vi "Configuration Tool Main.vi"() -> ()   [LabVIEW 2014, in "Advanced Configuration Tool.lvlib"]
doc: "This is the main VI for the configuration editor."
uses:
  Advanced Configuration Tool.lvlib
  Controls/StateCluster.ctl
  <vilib>/NI/Configuration Framework/Repository/NISE_CEF_Repository.lvclass
  <vilib>/NI/Configuration Framework/Node/NodeRef.ctl
  <vilib>/NI/Configuration Framework/Node/NISE_CEF_Node.lvclass
  <vilib>/NI/Configuration Framework/Node/UserEventRef.ctl
  <vilib>/NI/Configuration Framework/Controls/EventCluster.ctl
  Controls/AddMessage.ctl
  Controls/MoveMessage.ctl
  <vilib>/Utility/error.llb/DialogType.ctl
  <vilib>/NI/Configuration Framework/hierarchy repo/NISE_CEF_HierarchyRepo.lvclass
  Classes/My System/My System.lvclass
  <vilib>/NI/AMC/Read Termination Message.vi
  <vilib>/NI/AMC/Create Single Message.vi
  <vilib>/NI/AMC/Update Message Routing Info.vi
  <vilib>/NI/AMC/Globals.vi
  <vilib>/NI/AMC/Send Message.vi
  <vilib>/NI/AMC/AMC.lvlib
  <vilib>/NI/Configuration Framework/NISE_CEF_TreeControl.lvlib
  <vilib>/NI/Configuration Framework/serializable configuration/NISE_CEF_serializable configuration.lvclass
panel:
  in  "View":string(tree)
  in  "Exit":bool
  # "Configurator"
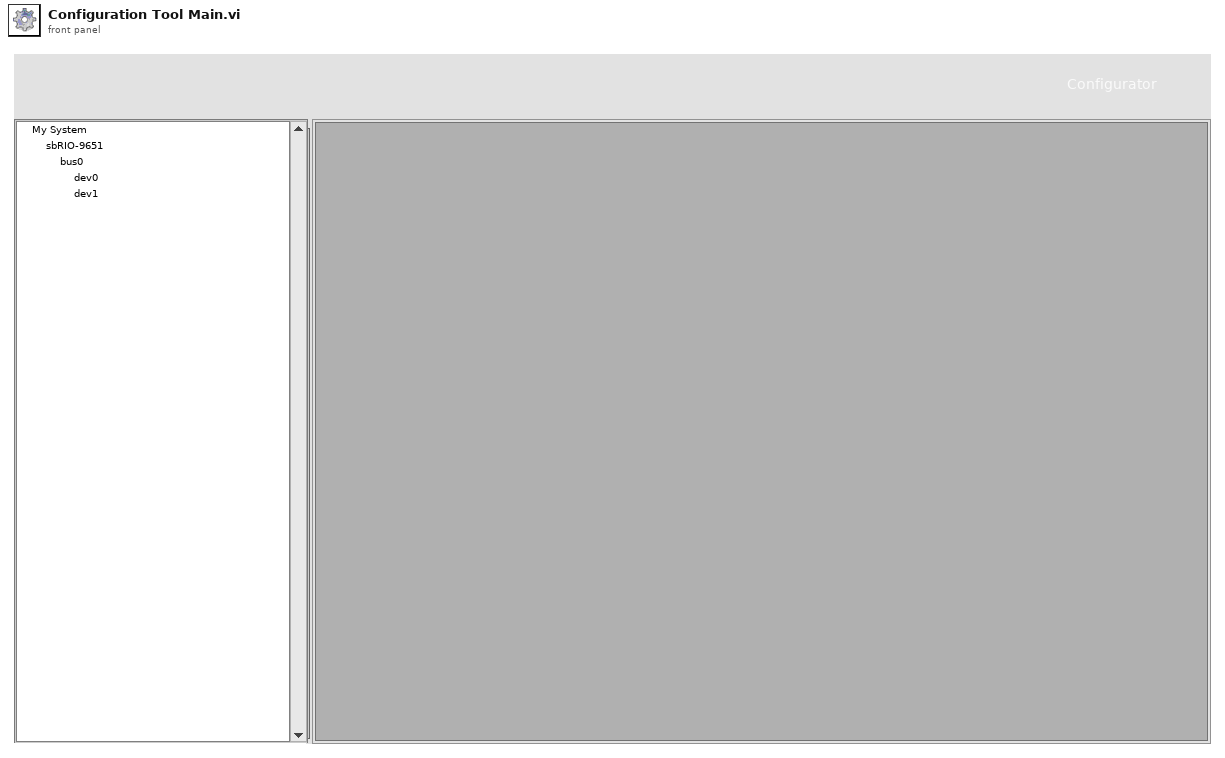
[diagram p1: front panel]
types:
  T1 = typedef "Advanced Configuration Tool.lvlib/StateCluster.ctl" = cluster{"repository":refnum<class "NISE_CEF_Repository.lvclass">, "root":T2, "unsaved changes":bool, "current path":path, "user event ref":T3, "glyph path":path, "classes path":path}
  T2 = typedef "NISE_CEF_Node.lvclass/NodeRef.ctl" = refnum<data-value>
  T3 = typedef "NISE_CEF_Node.lvclass/UserEventRef.ctl" = refnum<user-event>
  T4 = typedef "AMC.lvlib/Message Queue.ctl" = refnum<queue>
  T5 = typedef "Advanced Configuration Tool.lvlib/AddMessage.ctl" = cluster{"node type":string, "to add to":string}
  T6 = typedef "Advanced Configuration Tool.lvlib/MoveMessage.ctl" = cluster{"node ref":T2, "new parent":T2}
  T7 = typedef "NISE_CEF_TreeControl.lvlib/EventCluster.ctl" = cluster{"command":string, "data":string}
  T8 = typedef "Advanced Configuration Tool.lvlib/FilePaths.ctl" = cluster{"glyphs":path, "classes":path}
  T9 = typedef "DialogType.ctl" = u16
  T10 = typedef "NISE_CEF_Node.lvclass/Summary.ctl" = cluster{"ID":string, "parent ID":string, "node type":string, "text":string, "additional text":string, "glyph":string, "depth":i32}
  T11 = typedef "LVPoint32TypeDef.ctl" = cluster{"Horizontal":i32, "Vertical":i32}
  T12 = cluster{"data name":string, "drag data":variant}[]
  T13 = typedef "NISE_CEF_Node.lvclass/NodeMenuOptions.ctl" = cluster{"removable":bool, "movable":bool, "duplicate":bool}
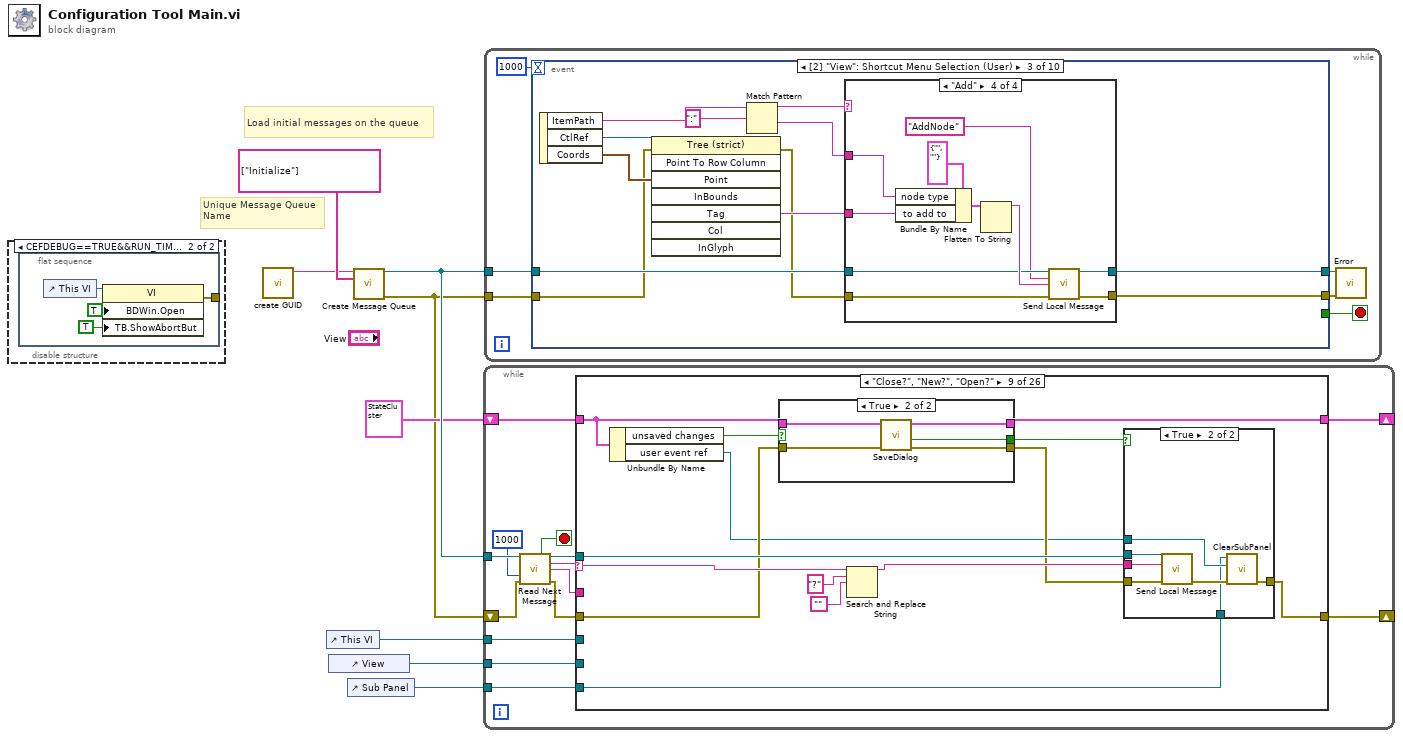
[diagram p0: block diagram]
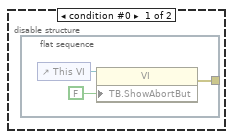
[diagram p2: hidden frame]
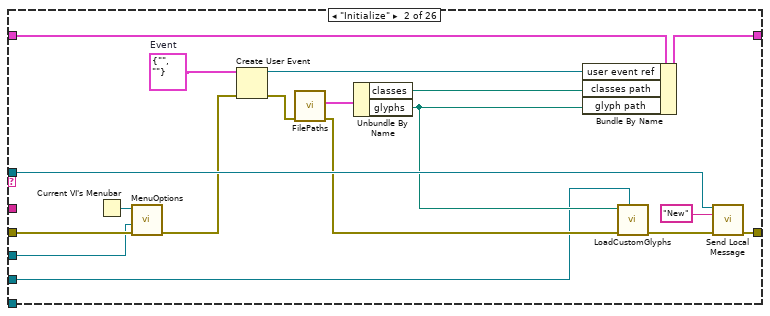
[diagram p4: hidden frame]
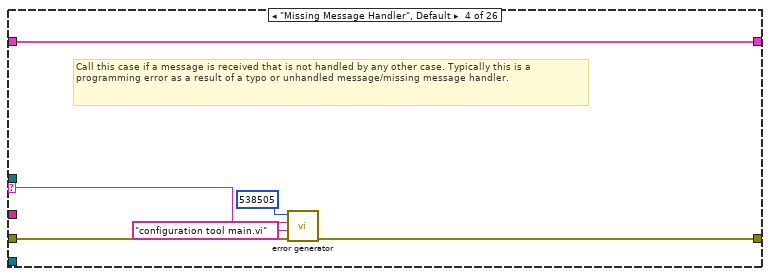
[diagram p6: hidden frame]
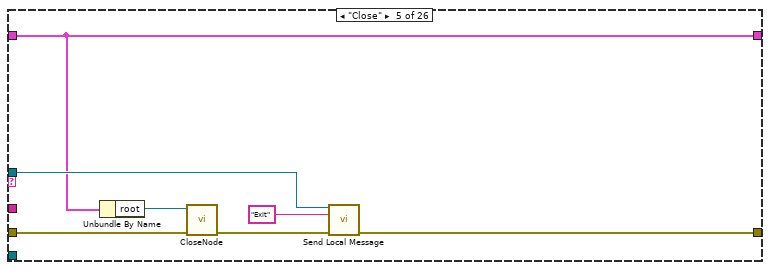
[diagram p7: hidden frame]
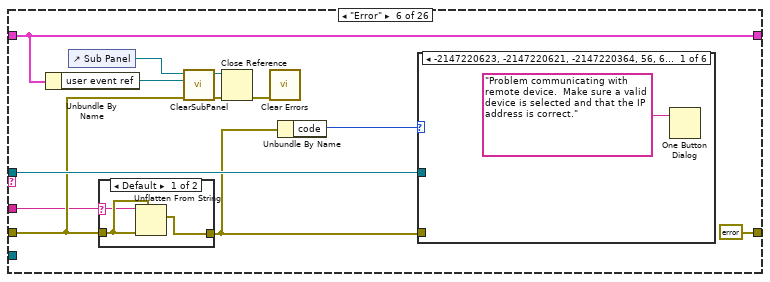
[diagram p8: hidden frame]
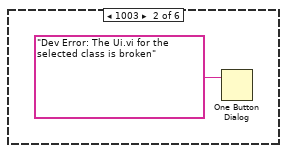
[diagram p10: hidden frame]
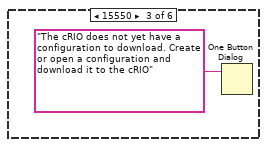
[diagram p11: hidden frame]
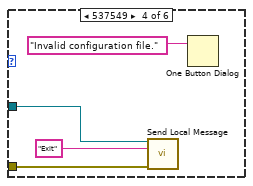
[diagram p12: hidden frame]
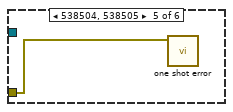
[diagram p13: hidden frame]
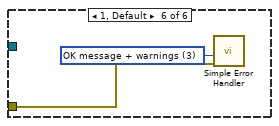
[diagram p14: hidden frame]
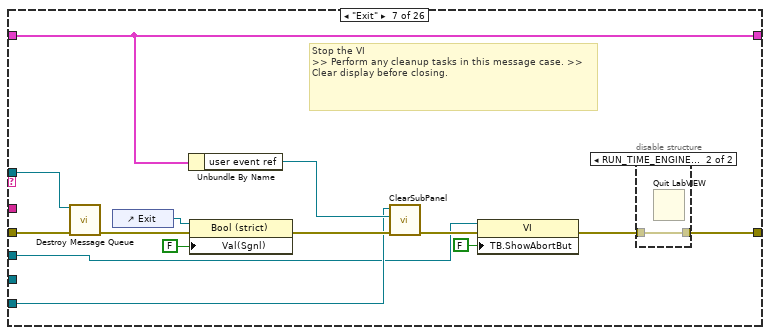
[diagram p15: hidden frame]
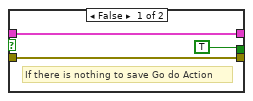
[diagram p18: hidden frame]
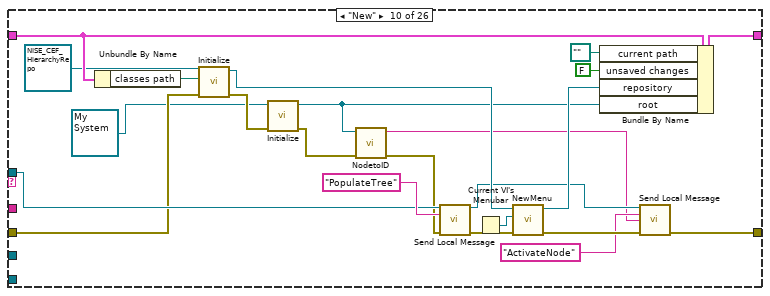
[diagram p20: hidden frame]
diagram:
  # "Unique Message Queue Name"
  # "Load initial messages on the queue"
  n1 = disable-structure shown="CEFDEBUG==TRUE&&RUN_TIME_ENGINE==False" {
    frame condition #0 {
      n2 = flat-sequence {
        tunnel: [w9] -> _
        frame #0 {
          n3 = control-ref of="This VI"() -> (w10:refnum<vi>)
          n4 = property class="VI"(reference=w10, "TB.ShowAbortBut"=FALSE ("Tool Bar:Show Abort Button")) -> (error out=w9:errorcluster)  [unwired: 1 in, 1 out]
        }
      }
    }
    frame condition #1 (active) {
      n5 = flat-sequence {
        tunnel: [w14] -> _
        frame #0 {
          n6 = control-ref of="This VI"() -> (w15:refnum<vi>)
          n7 = property class="VI"(reference=w15, "BDWin.Open"=TRUE ("Block Diagram Window:Open"), "TB.ShowAbortBut"=TRUE ("Tool Bar:Show Abort Button")) -> (error out=w14:errorcluster)  [unwired: 1 in, 1 out]
        }
      }
    }
  }
  n8 = call <vilib>:"create GUID.vi"() -> ("uuid"=w1:string)  [unwired: 11 in]
  n9 = control-ref of="This VI"() -> (w4:refnum<vi>)
  n10 = control-ref of="View"() -> (w3:refnum<vi>)
  n11 = control-ref of="Sub Panel"() -> (w2:refnum<vi>)
  n12 = call <vilib>:"Create Message Queue.vi"("message queue name"=w1, "initial message names"=string[] ["Initialize"]) -> ("message queue out"=w7:T4, "error out"=w5:errorcluster)  [unwired: 12 in]
  n13 = while "Message Processor" {
    shift-right: [w25] -> _
    shift-left: w5 -> [w24]
    tunnel: w7 -> [w23]
    shift-right: [w21] -> _
    shift-left: T1 {"repository"=refnum, "root"=refnum, "unsaved changes"=FALSE, "current path"=path "", "user event ref"=refnum, "glyph path"=path "", "classes path"=path ""} -> [w20]
    tunnel: w4 -> [w18]
    tunnel: w3 -> [w17]
    tunnel: w2 -> [w16]
    stop <- w29 stop-if-true
    n14 = call <vilib>:"Read Next Message.vi"("message queue in"=w23, "timeout (1 ms)"=1000, "error in"=w24) -> ("exit process?"=w29:bool, "message queue out"=w19:T4, "message name"=w28:string, "message value"=w27:string, "error out"=w26:errorcluster)  [unwired: 5 in, 3 out]
    n15 = case shown="\"Close?\", \"New?\", \"Open?\"" w28 {
      selector: w28 -> [_ _ _ w54 _ _ _ _ w118 _ _ _ _ _ _ _ _ _ _ w366 _ _ _ _ _ _]
      tunnel: w27 -> [_ _ _ _ _ w65 _ _ _ _ _ _ _ w240 w272 _ w300 w332 w346 w364 w404 w428 _ _ w471 w493]
      tunnel: w26 -> [w31 w49 w51 w56 w59 w68 w104 w108 w111 w155 w166 w206 w232 w247 w273 w290 w301 w322 w345 w369 w406 w427 w452 w461 w470 w491]
      tunnel: [w31 w45 w51 w55 w63 errorcluster {"status"=FALSE, "code"=0, "source"=""} ("error out") w97 w108 w122 w146 w162 w210 w234 w244 w260 w290 w304 w324 w349 w372 w410 w424 w447 w456 w467 w486] -> w25
      tunnel: [w30 w40 w50 w57 w61 w73 w96 w107 w113 w159 w167 w213 w233 w241 w269 w289 w307 w315 w342 w373 w408 w421 w454 w460 w465 w482] -> w21
      tunnel: w20 -> [w30 w41 w50 w57 w61 w73 w96 w107 w114 w158 w168 w208 w231 w242 w270 w289 w303 w320 w350 w373 w409 w429 w454 w460 w465 w494]
      tunnel: w19 -> [_ w44 _ _ w62 w76 w103 _ w121 w160 w164 w209 _ w243 w265 _ w291 _ _ w367 _ _ _ _ w466 w485]
      tunnel: w18 -> [_ w32 _ _ _ _ w92 _ _ _ _ _ _ _ _ _ _ _ _ _ _ _ w439 _ _ _]
      tunnel: w17 -> [_ w33 _ _ _ _ _ _ _ _ _ _ _ _ _ _ _ w316 w343 w361 w401 w422 w440 _ _ _]
      tunnel: w16 -> [_ _ _ _ _ _ w94 _ w109 _ _ _ _ _ _ _ _ _ _ _ _ _ w437 w455 w462 _]
      frame "------------Generic Operations------------" {
        # "Dummy case to add a seperation in the Case Structure menu"
      }
      frame "Initialize" {
        w35 = T7 {"command"="", "data"=""}  # Event
        n16 = Current VI's Menubar() -> (w48:refnum<k9>)
        n17 = call "MenuOptions.vi"("error in"=w49, "VI ref"=w32, "menu ref in"=w48) -> ("error out"=w39:errorcluster)  [unwired: 7 in, 1 out]
        n18 = Create User Event(user event datatype=w35, error in=w39) -> (user event=w34:refnum<user-event>, error out=w38:errorcluster)
        n19 = call "FilePaths.vi"("error in"=w38) -> ("error out"=w43:errorcluster, "paths"=w42:T8)  [unwired: 9 in]
        n20 = Unbundle By Name(w42) -> ("classes"=w37:path, "glyphs"=w36:path)
        n21 = Bundle By Name(cluster=w41, "user event ref"=w34, "classes path"=w37, "glyph path"=w36) -> (w40:T1)
        n22 = call <vilib>:"LoadCustomGlyphs.vi"("tree ref"=w33, "error in"=w43, "glyph directory"=w36) -> ("error out"=w46:errorcluster)  [unwired: 8 in]
        n23 = call <vilib>:"Send Local Message.vi"("message queue in"=w44, "message name"="New" ("Message Name"), "error in"=w46) -> ("error out"=w45:errorcluster)  [unwired: 10 in, 2 out]
      }
      frame "", "Idle" {
      }
      frame "Missing Message Handler", Default {
        # "Call this case if a message is received that is not handled by any other case. Typically this is a programming error as a result of a typo or unhandled message/missing message handler."
        n24 = call <vilib>:"error generator.vi"("error in"=w56, "source"="configuration tool main.vi", "append error message"=w54, "error code (0)"=538505) -> ("error out"=w55:errorcluster)  [unwired: 5 in]
      }
      frame "Close" {
        n25 = Unbundle By Name(w61) -> ("root"=w60:T2)
        n26 = call <vilib>:"CloseNode.vi"("error in"=w59, "node ref"=w60) -> ("error out"=w58:errorcluster)  [unwired: 9 in]
        n27 = call <vilib>:"Send Local Message.vi"("message queue in"=w62, "message name"="Exit", "error in"=w58) -> ("error out"=w63:errorcluster)  [unwired: 10 in, 2 out]
      }
      frame "Error" {
        n28 = Unbundle By Name(w73) -> ("user event ref"=w71:T3)
        n29 = control-ref of="Sub Panel"() -> (w72:refnum<vi>)
        n30 = case shown="Default" w65 {
          selector: w65 -> [w78 _]
          tunnel: w68 -> [w79 w80]
          tunnel: [w77 w80] -> w67
          frame Default {
            n31 = Unflatten From String(type=w79, binary string=w78, error in (no error)=w79) -> (value=w77:errorcluster)  [unwired: 2 in, 2 out]
          }
          frame "" {
          }
        }
        n32 = call <vilib>:"ClearSubPanel.vi"("error in"=w68, "user event ref"=w71, "sub panel ref in"=w72) -> ("error out"=w70:errorcluster, "sub panel ref out"=w69:refnum<vi>)  [unwired: 7 in]
        n33 = Close Reference(reference=w69, error in (no error)=w70) -> (error out=w66:errorcluster)
        n34 = call <vilib>:"Clear Errors.vi"("error in (no error)"=w66) -> ()  [unwired: 5 in, 2 out]
        n35 = Unbundle By Name(w67) -> ("code"=w74:i32)
        n36 = case shown="-2147220623, -2147220621, -2147220364, 56, 63" w74 {
          tunnel: w76 -> [_ _ _ w86 _ _]
          tunnel: w67 -> [_ _ _ w85 w88 w90]
          frame -2147220623, -2147220621, -2147220364, 56, 63 {
            n37 = One Button Dialog(message="Problem communicating with remote device.  Make sure a valid device is selected and that the IP address is correct.") -> ()  [unwired: 1 in, 1 out]
          }
          frame 1003 {
            n38 = One Button Dialog(message="Dev Error: The Ui.vi for the selected class is broken") -> ()  [unwired: 1 in, 1 out]
          }
          frame 15550 {
            n39 = One Button Dialog(message="The cRIO does not yet have a configuration to download. Create or open a configuration and download it to the cRIO") -> ()  [unwired: 1 in, 1 out]
          }
          frame 537549 {
            n40 = call <vilib>:"Send Local Message.vi"("message queue in"=w86, "message name"="Exit", "error in"=w85) -> ()  [unwired: 10 in, 3 out]
            n41 = One Button Dialog(message="Invalid configuration file.") -> ()  [unwired: 1 in, 1 out]
          }
          frame 538504, 538505 {
            n42 = call <vilib>:"one shot error.vi"("error in"=w88) -> ()  [unwired: 11 in]
          }
          frame 1, Default {
            w89 = T9 3 items=["no dialog", "OK message", "continue or stop message", "OK message + warnings", "continue/stop + warnings"] ("type of dialog (OK msg:1)")
            n43 = call <vilib>:"Simple Error Handler.vi"("type of dialog (OK msg:1)"=w89, "error in (no error)"=w90) -> ()  [unwired: 8 out]
          }
        }
      }
      frame "Exit" {
        # "Stop the VI                                                                             >> Perform any cleanup tasks in this message case. >> Clear display before closing."
        n44 = call <vilib>:"Destroy Message Queue.vi"("message queue in"=w103, "error in"=w104) -> ("error out"=w100:errorcluster)  [unwired: 11 in, 2 out]
        n45 = control-ref of="Exit"() -> (w102:refnum<vi>)
        n46 = Unbundle By Name(w96) -> ("user event ref"=w95:T3)
        n47 = property class="Bool (strict)"(reference=w102, error in=w100, "Val(Sgnl)"=FALSE ("Exit")) -> (error out=w99:errorcluster)  [unwired: 1 out]
        n48 = call <vilib>:"ClearSubPanel.vi"("error in"=w99, "user event ref"=w95, "sub panel ref in"=w94) -> ("error out"=w98:errorcluster)  [unwired: 7 in, 1 out]
        n49 = property class="VI"(reference=w92, error in=w98, "TB.ShowAbortBut"=FALSE ("Tool Bar:Show Abort Button")) -> (error out=w93:errorcluster)  [unwired: 1 out]
        n50 = disable-structure shown="RUN_TIME_ENGINE==True" {
          disable-tunnel: [w105 w106] -> w97
          disable-tunnel: w93 -> [w105 w106]
          frame condition #0 (active) {
          }
          frame condition #1 {
            n51 = Quit LabVIEW() -> ()  [unwired: 1 in]
          }
        }
      }
      frame "------------Menu Operations--------------" {
        # "Dummy case to add a seperation in the Case Structure menu"
      }
      frame "Close?", "New?", "Open?" {
        n52 = Unbundle By Name(w114) -> ("unsaved changes"=w116:bool, "user event ref"=w110:T3)
        n53 = case shown="True" w116 {
          tunnel: [TRUE ("SaveFlag") w130] -> w115
          tunnel: w114 -> [w124 w129]
          tunnel: [w124 w128] -> w113
          tunnel: w111 -> [w123 w127]
          tunnel: [w123 w126] -> w112
          frame False {
            # "If there is nothing to save Go do Action"
          }
          frame True {
            n54 = call "SaveDialog.vi"("error in"=w127, "state in"=w129) -> ("error out"=w126:errorcluster, "new"=w130:bool, "state out"=w128:T1)  [unwired: 7 in]
          }
        }
        n55 = Search and Replace String(input string=w118, search string="?", replace string="") -> (result string=w117:string)  [unwired: 5 in, 3 out]
        n56 = case shown="True" w115 {
          tunnel: w112 -> [w131 w138]
          tunnel: [w131 w134] -> w122
          tunnel: w121 -> [_ w137]
          tunnel: w117 -> [_ w136]
          tunnel: w110 -> [_ w133]
          tunnel: w109 -> [_ w132]
          frame False {
          }
          frame True {
            n57 = call <vilib>:"Send Local Message.vi"("message queue in"=w137, "message name"=w136, "error in"=w138) -> ("error out"=w135:errorcluster)  [unwired: 10 in, 2 out]
            n58 = call <vilib>:"ClearSubPanel.vi"("error in"=w135, "user event ref"=w133, "sub panel ref in"=w132) -> ("error out"=w134:errorcluster)  [unwired: 7 in, 1 out]
          }
        }
      }
      frame "New" {
        n59 = Unbundle By Name(w158) -> ("classes path"=w157:path)
        n60 = call-dynamic "Initialize.vi"("error in"=w155, "path"=w157, "repository in"=refnum<class "NISE_CEF_HierarchyRepo.lvclass"> refnum ("NISE_CEF_HierarchyRepo.lvclass")) -> ("error out"=w156:errorcluster, "repository out"=w149:refnum<class "NISE_CEF_HierarchyRepo.lvclass">)  [unwired: 7 in]
        n61 = call-dynamic "Initialize.vi"("error in"=w156, "node in"=refnum<class "My System.lvclass"> refnum ("My System.lvclass")) -> ("error out"=w143:errorcluster, "data value reference"=w144:T2)  [unwired: 7 in, 1 out]
        n62 = call <vilib>:"NodetoID.vi"("error in"=w143, "node ref"=w144) -> ("error out"=w142:errorcluster, "ID"=w140:string)  [unwired: 8 in]
        n63 = call <vilib>:"Send Local Message.vi"("message queue in"=w160, "message name"="PopulateTree", "error in"=w142) -> ("message queue out"=w145:T4, "error out"=w151:errorcluster)  [unwired: 10 in, 1 out]
        n64 = Current VI's Menubar() -> (w150:refnum<k9>)
        n65 = call <vilib>:"NewMenu.vi"("error in"=w151, "menu ref in"=w150, "NISE_CEF_Repository in"=w149) -> ("error out"=w147:errorcluster, "NISE_CEF_Repository out"=w148:refnum<class "NISE_CEF_HierarchyRepo.lvclass">)  [unwired: 6 in, 1 out]
        n66 = Bundle By Name(cluster=w158, "current path"=path "", "unsaved changes"=FALSE, "repository"=w148, "root"=w144) -> (w159:T1)
        n67 = call <vilib>:"Send Local Message.vi"("message queue in"=w145, "message name"="ActivateNode", "message value"=w140, "error in"=w147) -> ("error out"=w146:errorcluster)  [unwired: 9 in, 2 out]
      }
      frame "Open" {
        n68 = in-place {
          in-place-border: w166 -> [w174]
          in-place-border: [w173] -> w163
          n69 = in-place-cluster #1(w168) -> ("current path"=w170:path, "repository"=w182:refnum<class "NISE_CEF_Repository.lvclass">, "root"=w178:T2)  [unwired: 1 out]
          n70 = call "generate default path.vi"("current file path"=w170) -> ("browse path"=w169:path)  [unwired: 10 in]
          n71 = call "FileDialog.vi"("error in"=w174, "start path"=w169) -> ("error out"=w175:errorcluster, "cancelled"=w176:bool, "selected path"=w172:path)  [unwired: 7 in]
          n72 = Compound Arithmetic op=OR(invert w176) -> (w177:bool)
          n73 = case shown="True" w177 {
            tunnel: w182 -> [w183 w195]
            tunnel: [w183 w193] -> w180
            tunnel: [w184 w191] -> w173
            tunnel: [w185 w190] -> w179
            tunnel: w172 -> [_ w188]
            tunnel: w175 -> [w184 w187]
            tunnel: w178 -> [w185 w186]
            frame False {
            }
            frame True {
              n74 = call-dynamic "Open.vi"("error in"=w187, "file path"=w188, "repository in"=w195) -> ("error out"=w192:errorcluster, "invalid?"=w189:bool, "repository out"=w194:refnum<class "NISE_CEF_Repository.lvclass">)  [unwired: 6 in]
              n75 = case shown="False" w189 {
                tunnel: w194 -> [w200 w203]
                tunnel: [w199 w203] -> w193
                tunnel: w192 -> [w198 w202]
                tunnel: [w197 w202] -> w191
                tunnel: [w196 w201] -> w190
                tunnel: w186 -> [_ w201]
                frame False {
                  n76 = call-dynamic "WriteTree.vi"("error in"=w198, "repository in"=w200) -> ("error out"=w197:errorcluster, "root"=w196:T2, "repository out"=w199:refnum<class "NISE_CEF_Repository.lvclass">)  [unwired: 7 in]
                }
                frame True {
                }
              }
            }
          }
          n77 = Select(t=w170, s=w173, f=w172) -> (s? t:f=w171:path)
          n78 = in-place-cluster #1("current path"=w171, "unsaved changes"=FALSE ("SaveFlag"), "repository"=w180, "root"=w179) -> (w167:T1)
        }
        n79 = call <vilib>:"Send Local Message.vi"("message queue in"=w164, "message name"="PopulateTree", "error in"=w163) -> ("error out"=w162:errorcluster)  [unwired: 10 in, 2 out]
      }
      frame "Save" {
        n80 = in-place {
          in-place-border: w206 -> [w218]
          in-place-border: [w217] -> w205
          in-place-border: [w215] -> w204
          n81 = in-place-cluster #2(w208) -> ("current path"=w216:path, "root"=w219:T2, "repository"=w220:refnum<class "NISE_CEF_Repository.lvclass">)
          n82 = Empty String/Path?(string/path=w216) -> (empty?=w215:bool)
          n83 = call-dynamic "ReadTree.vi"("error in"=w218, "root"=w219, "repository in"=w220) -> ("error out"=w217:errorcluster, "repository out"=w214:refnum<class "NISE_CEF_Repository.lvclass">)  [unwired: 7 in]
          n84 = in-place-cluster #2("current path"=w216, "root"=w219, "repository"=w214) -> (w207:T1)
        }
        n85 = case shown="True" w204 {
          tunnel: w207 -> [w224 w226]
          tunnel: [w223 w225] -> w213
          tunnel: [w222 w227] -> w211
          tunnel: w205 -> [w221 w228]
          frame False {
            n86 = call "Save.vi"("error in"=w221, "state in"=w224) -> ("error out"=w222:errorcluster, "state out"=w223:T1)  [unwired: 8 in]
          }
          frame True {
            # "Empty path use Dialog"
            n87 = call "SaveAs.vi"("error in"=w228, "state in"=w226) -> ("error out"=w227:errorcluster, "state out"=w225:T1)  [unwired: 7 in, 1 out]
          }
        }
        n88 = call <vilib>:"Send Local Message.vi"("message queue in"=w209, "message name"="PopulateTree", "error in"=w211) -> ("error out"=w210:errorcluster)  [unwired: 10 in, 2 out]
      }
      frame "SaveAs" {
        n89 = in-place {
          in-place-border: w232 -> [w236]
          in-place-border: [w235] -> w230
          n90 = in-place-cluster #3(w231) -> ("root"=w237:T2, "repository"=w239:refnum<class "NISE_CEF_Repository.lvclass">)
          n91 = call-dynamic "ReadTree.vi"("error in"=w236, "root"=w237, "repository in"=w239) -> ("error out"=w235:errorcluster, "repository out"=w238:refnum<class "NISE_CEF_Repository.lvclass">)  [unwired: 7 in]
          n92 = in-place-cluster #3("root"=w237, "repository"=w238) -> (w229:T1)
        }
        n93 = call "SaveAs.vi"("error in"=w230, "state in"=w229) -> ("error out"=w234:errorcluster, "state out"=w233:T1)  [unwired: 7 in, 1 out]
      }
      frame "Custom View" {
        n94 = in-place {
          in-place-border: w247 -> [w258]
          in-place-border: [w257] -> w245
          in-place-border: w240 -> [w248]
          n95 = in-place-cluster #4(w242) -> ("repository"=w252:refnum<class "NISE_CEF_Repository.lvclass">, "root"=w251:T2)
          n96 = call-dynamic "ReadTree.vi"("error in"=w258, "root"=w251, "repository in"=w252) -> ("error out"=w255:errorcluster, "repository out"=w254:refnum<class "NISE_CEF_Repository.lvclass">)  [unwired: 7 in]
          n97 = call-dynamic "CustomView.vi"("error in"=w255, "view name"=w248, "repository in"=w254) -> ("error out"=w256:errorcluster, "repository out"=w253:refnum<class "NISE_CEF_Repository.lvclass">)  [unwired: 7 in]
          n98 = call-dynamic "WriteTree.vi"("error in"=w256, "repository in"=w253) -> ("error out"=w257:errorcluster, "root"=w249:T2, "repository out"=w250:refnum<class "NISE_CEF_Repository.lvclass">)  [unwired: 7 in]
          n99 = in-place-cluster #4("repository"=w250, "root"=w249) -> (w241:T1)
        }
        n100 = call <vilib>:"Send Local Message.vi"("message queue in"=w243, "message name"="PopulateTree", "error in"=w245) -> ("error out"=w244:errorcluster)  [unwired: 10 in, 2 out]
      }
      frame "CustomFileMenu" {
        n101 = Unflatten From String(type=cluster{"ItemTag":string, string} {"ItemTag"="", ""} ("output cluster"), binary string=w272, error in (no error)=w273) -> (value=w259:cluster{"ItemTag":string, string}, error out=w268:errorcluster)  [unwired: 2 in, 1 out]
        n102 = Unbundle By Name(w270) -> ("repository"=w267:refnum<class "NISE_CEF_Repository.lvclass">)
        n103 = Unbundle(w259) -> ("ItemTag"=w264:string, w263:string)
        n104 = call-dynamic "HandleMenu.vi"("message queue"=w265, "error in"=w268, "Item Path"=w263, "ItemTag"=w264, "NISE_CEF_Repository in"=w267) -> ("error out"=w262:errorcluster, "handled?"=w261:bool, "NISE_CEF_Repository out"=w266:refnum<class "NISE_CEF_Repository.lvclass">)  [unwired: 4 in]
        n105 = case shown="False" w261 {
          tunnel: w262 -> [w277 w288]
          tunnel: [w278 w288] -> w260
          tunnel: w259 -> [w276 _]
          frame False {
            n106 = Unbundle(w276) -> ("ItemTag"=w275:string, w274:string)
            n107 = disable-structure shown="Default" {
              disable-tunnel: w277 -> [w284 w287]
              disable-tunnel: [w283 w287] -> w278
              disable-tunnel: w274 -> [w282 _]
              disable-tunnel: w275 -> [w281 _]
              frame condition #0 (active) {
                n108 = Concatenate Strings(w281, "::" ("string"), w282) -> (w280:string)
                n109 = call <vilib>:"error generator.vi"("error in"=w284, "source"="configuration tool main.vi", "append error message"=w280, "error code (0)"=538506) -> ("error out"=w283:errorcluster)  [unwired: 5 in]
              }
              frame condition #1 {
              }
            }
          }
          frame True {
          }
        }
        n110 = Bundle By Name(cluster=w270, "repository"=w266) -> (w269:T1)
      }
      frame "-------TreeControl Operations-----------" {
        # "Dummy case to add a seperation in the Case Structure menu"
      }
      frame "Select Target" {
        n111 = in-place {
          in-place-border: w301 -> [w311]
          in-place-border: w300 -> [w310]
          in-place-border: [w309] -> w297
          in-place-border: [w308] -> w298
          n112 = in-place-cluster #5(w303) -> ("repository"=w313:refnum<class "NISE_CEF_Repository.lvclass">)
          n113 = call-dynamic "GetClassPath.vi"("error in"=w311, "class name"=w310, "Repository in"=w313) -> ("error out"=w309:errorcluster, "class path"=w308:path, "Repository out"=w312:refnum<class "NISE_CEF_Repository.lvclass">)  [unwired: 6 in]
          n114 = in-place-cluster #5("repository"=w312) -> (w302:T1)
        }
        n115 = call <vilib>:"Get LV Class Default Value.vi"("error in (no error)"=w297, "class path"=w298) -> ("error out"=w296:errorcluster, "object"=w299:refnum<class>)  [unwired: 8 in]
        n116 = To More Specific Class(target class=refnum<class "NISE_CEF_Node.lvclass"> refnum ("Node.lvclass"), reference=w299, error in=w296) -> (specific class reference=w294:refnum<class "NISE_CEF_Node.lvclass">, error out=w293:errorcluster)
        n117 = call-dynamic "Initialize.vi"("error in"=w293, "node in"=w294) -> ("error out"=w292:errorcluster, "data value reference"=w306:T2)  [unwired: 7 in, 1 out]
        n118 = Bundle By Name(cluster=w302, "root"=w306) -> (w307:T1)
        n119 = call <vilib>:"Send Local Message.vi"("message queue in"=w291, "message name"="PopulateTree", "error in"=w292) -> ("error out"=w304:errorcluster)  [unwired: 10 in, 2 out]
      }
      frame "AddNode" {
        n120 = Unflatten From String(type=T5 {"node type"="", "to add to"=""} ("input cluster"), binary string=w332) -> (value=w330:T5)  [unwired: 3 in, 2 out]
        n121 = Unbundle By Name(w330) -> ("to add to"=w327:string, "node type"=w318:string)
        n122 = in-place {
          in-place-border: w322 -> [w338]
          in-place-border: [w337] -> w321
          in-place-border: w318 -> [w336]
          in-place-border: [w335] -> w317
          n123 = in-place-cluster #6(w320) -> ("repository"=w340:refnum<class "NISE_CEF_Repository.lvclass">)
          n124 = call-dynamic "GetClassPath.vi"("error in"=w338, "class name"=w336, "Repository in"=w340) -> ("error out"=w337:errorcluster, "class path"=w335:path, "Repository out"=w339:refnum<class "NISE_CEF_Repository.lvclass">)  [unwired: 6 in]
          n125 = in-place-cluster #6("repository"=w339) -> (w319:T1)
        }
        n126 = call <vilib>:"Get LV Class Default Value.vi"("error in (no error)"=w321, "class path"=w317) -> ("error out"=w333:errorcluster, "object"=w334:refnum<class>)  [unwired: 8 in]
        n127 = To More Specific Class(target class=refnum<class "NISE_CEF_Node.lvclass"> refnum ("Node.lvclass"), reference=w334, error in=w333) -> (specific class reference=w329:refnum<class "NISE_CEF_Node.lvclass">, error out=w326:errorcluster)
        n128 = call <vilib>:"AddNode.vi"("error in"=w326, "node in"=w329, "parent node ID"=w327) -> ("error out"=w325:errorcluster, "summary"=w323:T10[])  [unwired: 7 in]
        n129 = Bundle By Name(cluster=w319, "unsaved changes"=TRUE) -> (w315:T1)
        n130 = call <vilib>:"PopulateTreeSumary.vi"("error in"=w325, "array"=w323, "tree ref in"=w316) -> ("error out"=w324:errorcluster)  [unwired: 8 in]
      }
      frame "Duplicate" {
        n131 = call <vilib>:"IDtoNode.vi"("error in"=w345, "ID"=w346) -> ("error out"=w347:errorcluster, "invalid Id"=w344:bool, "node ref"=w348:T2)  [unwired: 7 in]
        n132 = case shown="False" w344 {
          tunnel: [w359 w360] -> w349
          tunnel: w348 -> [w358 _]
          tunnel: w347 -> [w355 w360]
          tunnel: w343 -> [w351 _]
          frame False {
            n133 = call <vilib>:"DuplicateNode.vi"("same parent?"=TRUE ("s"), "error in"=w355, "node ref in"=w358) -> ("error out"=w356:errorcluster, "new node ref"=w357:T2)  [unwired: 7 in]
            n134 = call <vilib>:"Summary.vi"("error in"=w356, "node self ref"=w357) -> ("error out"=w353:errorcluster, "summary"=w352:T10[])  [unwired: 8 in]
            n135 = call <vilib>:"PopulateTreeSumary.vi"("error in"=w353, "array"=w352, "tree ref in"=w351) -> ("error out"=w359:errorcluster)  [unwired: 8 in]
          }
          frame True {
          }
        }
        n136 = Bundle By Name(cluster=w350, "unsaved changes"=TRUE) -> (w342:T1)
      }
      frame "CustomMenuAction" {
        n137 = Match Pattern(string=w364, regular expression=":") -> (before substring=w363:string, after substring=w362:string)  [unwired: 1 in, 2 out]
        n138 = call <vilib>:"IDtoNode.vi"("error in"=w369, "ID"=w362) -> ("error out"=w370:errorcluster, "invalid Id"=w368:bool, "node ref"=w371:T2)  [unwired: 7 in]
        n139 = case shown="False" w368 {
          tunnel: [w376 w400] -> w372
          tunnel: w371 -> [w381 _]
          tunnel: w370 -> [w379 w400]
          tunnel: w367 -> [w380 _]
          tunnel: w366 -> [_ _]
          tunnel: w363 -> [w377 _]
          tunnel: w361 -> [w374 _]
          frame False {
            n140 = in-place {
              in-place-border: w380 -> [w398]
              in-place-border: w379 -> [w396]
              in-place-border: [w395] -> w375
              in-place-border: [w394] -> w378
              in-place-border: w377 -> [w393]
              in-place-border: w374 -> [w392]
              n141 = in-place-dvr #7(w381) -> (w399:refnum<class "NISE_CEF_Node.lvclass">)  [unwired: 1 out]
              n142 = call-dynamic "MenuHandler.vi"("tree control"=w392, "main message queue"=w398, "error in"=w396, "menu string"=w393, "NISE_CEF_Node in"=w399) -> ("error out"=w395:errorcluster, "Unhandled"=w394:bool, "NISE_CEF_Node out"=w397:refnum<class "NISE_CEF_Node.lvclass">)  [unwired: 4 in]
              n143 = in-place-dvr #7(w397) -> ()  [unwired: 2 out]
            }
            n144 = case shown="False" w378 {
              tunnel: w377 -> [_ w383]
              tunnel: [w382 w384] -> w376
              tunnel: w375 -> [w382 w385]
              frame False {
              }
              frame True {
                n145 = disable-structure shown="CEFDEBUG==TRUE" {
                  disable-tunnel: w385 -> [w388 w391]
                  disable-tunnel: [w387 w391] -> w384
                  disable-tunnel: w383 -> [w386 _]
                  frame condition #0 (active) {
                    n146 = call <vilib>:"error generator.vi"("error in"=w388, "source"="configuration tool main.vi", "append error message"=w386, "error code (0)"=538506) -> ("error out"=w387:errorcluster)  [unwired: 5 in]
                  }
                  frame condition #1 {
                  }
                }
              }
            }
          }
          frame True {
          }
        }
      }
      frame "RefreshNode" {
        # "Refreshes the node in the Tree               Sets the save flag to true                       This case can be called from the UIs of the nodes"
        n147 = call <vilib>:"IDtoNode.vi"("error in"=w406, "ID"=w404) -> ("error out"=w405:errorcluster, "invalid Id"=w402:bool, "node ref"=w403:T2)  [unwired: 7 in]
        n148 = case shown="False" w402 {
          tunnel: [w417 w419] -> w410
          tunnel: w405 -> [w413 w419]
          tunnel: w403 -> [w412 _]
          tunnel: w401 -> [w411 _]
          frame False {
            n149 = call <vilib>:"Summary.vi"("error in"=w413, "node self ref"=w412) -> ("error out"=w415:errorcluster, "summary"=w414:T10[])  [unwired: 8 in]
            n150 = call <vilib>:"RefreshSubTree.vi"("error in"=w415, "node information"=w414, "tree ref in"=w411) -> ("error out"=w418:errorcluster, "tree ref out"=w416:refnum<vi>)  [unwired: 7 in]
            n151 = Close Reference(reference=w416, error in (no error)=w418) -> (error out=w417:errorcluster)
          }
          frame True {
          }
        }
        n152 = Bundle By Name(cluster=w409, "unsaved changes"=TRUE ("SaveFlag")) -> (w408:T1)
      }
      frame "RemoveNode" {
        n153 = call <vilib>:"IDtoNode.vi"("error in"=w427, "ID"=w428) -> ("error out"=w426:errorcluster, "invalid Id"=w423:bool, "node ref"=w425:T2)  [unwired: 7 in]
        n154 = case shown="False" w423 {
          tunnel: w426 -> [w435 w436]
          tunnel: w425 -> [w434 _]
          tunnel: [w431 w436] -> w424
          tunnel: w422 -> [w430 _]
          frame False {
            n155 = call <vilib>:"RemoveNode.vi"("error in"=w435, "node"=w434) -> ("error out"=w432:errorcluster, "node ID"=w433:string)  [unwired: 8 in]
            n156 = call <vilib>:"ClearTreeNode.vi"("error in"=w432, "tag"=w433, "tree reference"=w430) -> ("error out"=w431:errorcluster)  [unwired: 8 in]
          }
          frame True {
          }
        }
        n157 = Bundle By Name(cluster=w429, "unsaved changes"=TRUE) -> (w421:T1)
      }
      frame "PopulateTree" {
        n158 = Unbundle By Name(w454) -> ("current path"=w445:path, "user event ref"=w446:T3, "root"=w450:T2)
        n159 = call <vilib>:"Summary.vi"("error in"=w452, "depth"=0 ("Depth"), "node self ref"=w450) -> ("error out"=w451:errorcluster, "summary"=w453:T10[])  [unwired: 7 in]
        n160 = call <vilib>:"Check if File or Folder Exists.vi"("path"=w445) -> ("file or folder exists?"=w443:bool, "dup path"=w444:path)  [unwired: 8 in, 1 out]
        n161 = Strip Path(path=w444) -> (name=w442:string)  [unwired: 1 out]
        n162 = call <vilib>:"RefreshEntireTree.vi"("calling VI in"=w439, "error in"=w451, "array"=w453, "tree ref in"=w440) -> ("error out"=w448:errorcluster)  [unwired: 7 in]
        n163 = Select(t=w442, s=w443, f="Advanced Configurator Sample Project") -> (s? t:f=w438:string)
        n164 = property class="VI"(reference=w439, "Front Panel.Title"=w438) -> ()  [unwired: 1 in, 2 out]
        n165 = call <vilib>:"ClearSubPanel.vi"("error in"=w448, "user event ref"=w446, "sub panel ref in"=w437) -> ("error out"=w447:errorcluster)  [unwired: 7 in, 1 out]
      }
      frame "CleansubPanel" {
        n166 = Unbundle By Name(w460) -> ("user event ref"=w459:T3)
        n167 = call <vilib>:"ClearSubPanel.vi"("error in"=w461, "user event ref"=w459, "sub panel ref in"=w455) -> ("error out"=w458:errorcluster, "sub panel ref out"=w457:refnum<vi>)  [unwired: 7 in]
        n168 = Close Reference(reference=w457, error in (no error)=w458) -> (error out=w456:errorcluster)
      }
      frame "ActivateNode" {
        n169 = Unbundle By Name(w465) -> ("user event ref"=w464:T3)
        n170 = call <vilib>:"IDtoNode.vi"("error in"=w470, "ID"=w471) -> ("error out"=w463:errorcluster, "invalid Id"=w469:bool, "node ref"=w468:T2)  [unwired: 7 in]
        n171 = case shown="False" w469 {
          tunnel: w468 -> [w478 _]
          tunnel: [w479 w480] -> w467
          tunnel: w463 -> [w476 w480]
          tunnel: w466 -> [w474 _]
          tunnel: w464 -> [w475 _]
          tunnel: w462 -> [w472 _]
          frame False {
            n172 = call <vilib>:"ClearSubPanel.vi"("error in"=w476, "user event ref"=w475, "sub panel ref in"=w472) -> ("error out"=w477:errorcluster, "sub panel ref out"=w473:refnum<vi>)  [unwired: 7 in]
            n173 = call <vilib>:"LoadNodeUI.vi"("user event out"=w475, "error in"=w477, "sub panel ref in"=w473, "main queue"=w474, "node"=w478) -> ("error out"=w479:errorcluster)  [unwired: 6 in]
          }
          frame True {
          }
        }
      }
      frame "Move" {
        n174 = Unflatten From String(type=T6 {"node ref"=refnum, "new parent"=refnum} ("Cluster"), binary string=w493, error in (no error)=w491) -> (value=w490:T6, error out=w489:errorcluster)  [unwired: 2 in, 1 out]
        n175 = Unbundle By Name(w490) -> ("node ref"=w484:T2, "new parent"=w483:T2)
        n176 = call <vilib>:"MoveNode.vi"("error in"=w489, "new parent"=w483, "node"=w484) -> ("error out"=w487:errorcluster)  [unwired: 8 in]
        n177 = Bundle By Name(cluster=w494, "unsaved changes"=TRUE) -> (w482:T1)
        n178 = call <vilib>:"Send Local Message.vi"("message queue in"=w485, "message name"="PopulateTree", "error in"=w487) -> ("error out"=w486:errorcluster)  [unwired: 10 in, 2 out]
      }
    }
  }
  n179 = while "User Interface Event Handler" {
    tunnel: w7 -> [w499]
    tunnel: w5 -> [w495]
    stop <- w498 stop-if-true
    n180 = event shown="[2] \"View\": Shortcut Menu Selection (User)" {
      selector: _ -> [_ _ _ _ _ _ _ _ _ _]
      dyn-events: _ -> [_ _ _ _ _ _ _ _ _ _]
      timeout: 1000 -> [_ _ _ _ _ _ _ _ _ _]
      tunnel: w499 -> [w502 w511 w536 w588 w616 w623 w652 w656 w666 w672]
      tunnel: [_ _ _ _ TRUE _ _ _ _ _] -> w498
      tunnel: [w502 w511 w533 w586 w612 w623 w649 w656 w664 w671] -> w497
      tunnel: [w501 w507 w532 w585 w613 w619 w648 w653 w662 w669] -> w496
      tunnel: w495 -> [w501 w510 w531 w587 w614 w622 w647 w655 w663 w670]
      event Timeout {
        # "Timeout code can be added here for autosave or Lock Screen"
        n181 = event-data() -> ()  [unwired: 1 in, 1 out]
      }
      event "View": Shortcut Menu Activation? {
        n182 = event-data() -> ("CtlRef"=w517:refnum<vi>, "Coords"=w516:T11, "MenuRef"=w513:refnum<k9>)  [unwired: 1 in]
        n183 = invoke class="Tree (strict)" method="Point To Row Column"(reference=w517, error in=w510, "Point"=w516) -> (error out=w509:errorcluster, "Tag"=w515:string)  [unwired: 5 in, 6 out]
        n184 = call <vilib>:"IDtoNode.vi"("error in"=w509, "ID"=w515) -> ("error out"=w505:errorcluster, "invalid Id"=w512:bool, "node ref"=w514:T2)  [unwired: 7 in]
        n185 = case shown="False" w512 {
          selector: w512 -> [_ w528]
          tunnel: w514 -> [w522 _]
          tunnel: w513 -> [w521 _]
          tunnel: [w520 _] -> w508
          tunnel: [w519 _] -> w506
          tunnel: w505 -> [w518 w529]
          tunnel: [w518 w529] -> w504
          tunnel: [_ w528] -> w503
          frame False {
            n186 = in-place {
              in-place-border: w521 -> [w525]
              in-place-border: [w523] -> w520
              n187 = in-place-dvr #8(w522) -> (w527:refnum<class "NISE_CEF_Node.lvclass">, w524:errorcluster)
              n188 = call-dynamic "ShortcutMenu.vi"("error in"=w524, "menu ref in"=w525, "node in"=w527) -> ("error out"=w523:errorcluster, "node out"=w526:refnum<class "NISE_CEF_Node.lvclass">)  [unwired: 6 in, 1 out]
              n189 = in-place-dvr #8(w526) -> (w519:errorcluster)  [unwired: 1 out]
            }
          }
          frame True {
          }
        }
        n190 = Merge Errors(w506, w508, w504) -> (w507:errorcluster)
        n191 = event-data("Discard?"=w503) -> ()  [unwired: 1 in, 1 out]
      }
      event "View": Shortcut Menu Selection (User) {
        n192 = event-data() -> ("ItemPath"=w535:string, "CtlRef"=w539:refnum<vi>, "Coords"=w540:T11)  [unwired: 1 in]
        n193 = invoke class="Tree (strict)" method="Point To Row Column"(reference=w539, error in=w531, "Point"=w540) -> (error out=w530:errorcluster, "Tag"=w534:string)  [unwired: 5 in, 6 out]
        n194 = Match Pattern(string=w535, regular expression=":") -> (before substring=w538:string, after substring=w537:string)  [unwired: 1 in, 2 out]
        n195 = case shown="\"Add\"" w538 {
          selector: w538 -> [w543 _ _ _]
          tunnel: w537 -> [_ _ _ w567]
          tunnel: w536 -> [w549 w556 w562 w569]
          tunnel: w534 -> [w545 w554 w560 w568]
          tunnel: [w546 w553 w559 w565] -> w533
          tunnel: [w547 w552 w557 w563] -> w532
          tunnel: w530 -> [w548 w551 w558 w564]
          frame Default {
            n196 = Concatenate Strings(w543, ":" ("string"), w545) -> (w542:string)
            n197 = call <vilib>:"Send Local Message.vi"("message queue in"=w549, "message name"="CustomMenuAction" ("Message Name"), "message value"=w542, "error in"=w548) -> ("message queue out"=w546:T4, "error out"=w547:errorcluster)  [unwired: 9 in, 1 out]
          }
          frame "Remove" {
            n198 = call <vilib>:"Send Local Message.vi"("message queue in"=w556, "message name"="RemoveNode" ("Message Name"), "message value"=w554, "error in"=w551) -> ("message queue out"=w553:T4, "error out"=w552:errorcluster)  [unwired: 9 in, 1 out]
          }
          frame "Duplicate" {
            n199 = call <vilib>:"Send Local Message.vi"("message queue in"=w562, "message name"="Duplicate" ("Message Name"), "message value"=w560, "error in"=w558) -> ("message queue out"=w559:T4, "error out"=w557:errorcluster)  [unwired: 9 in, 1 out]
          }
          frame "Add" {
            n200 = Bundle By Name(cluster=T5 {"node type"="", "to add to"=""} ("input cluster"), "node type"=w567, "to add to"=w568) -> (w570:T5)
            n201 = Flatten To String(anything=w570) -> (data string=w571:string)  [unwired: 3 in, 2 out]
            n202 = call <vilib>:"Send Local Message.vi"("message queue in"=w569, "message name"="AddNode" ("Message Name"), "message value"=w571, "error in"=w564) -> ("message queue out"=w565:T4, "error out"=w563:errorcluster)  [unwired: 9 in, 1 out]
          }
        }
      }
      event "View": Drop {
        n203 = event-data() -> ("CtlRef"=w591:refnum<vi>, "Coords"=w590:T11)  [unwired: 1 in]
        n204 = invoke class="Tree (strict)" method="Point To Row Column"(reference=w591, error in=w587, "Point"=w590) -> (reference out=w589:refnum<vi>, error out=w584:errorcluster, "Tag"=w581:string)  [unwired: 5 in, 5 out]
        n205 = call <vilib>:"ValidDragDrop.vi"("error in"=w584, "drag over"=w581, "tree ref in"=w589) -> ("error out"=w576:errorcluster, "accepted"=w579:bool, "drag"=w583:string, "tree ref out"=w593:refnum<vi>)  [unwired: 5 in]
        n206 = call <vilib>:"IDtoNode.vi"("error in"=w576, "ID"=w581) -> ("error out"=w577:errorcluster, "invalid Id"=w574:bool, "node ref"=w580:T2)  [unwired: 7 in]
        n207 = call <vilib>:"IDtoNode.vi"("error in"=w577, "ID"=w583) -> ("error out"=w575:errorcluster, "invalid Id"=w573:bool, "node ref"=w582:T2)  [unwired: 7 in]
        n208 = Compound Arithmetic op=AND(w579, invert w574, invert w573) -> (w578:bool)
        n209 = case shown="True" w578 {
          tunnel: w583 -> [_ w609]
          tunnel: w593 -> [_ w611]
          tunnel: [_ TRUE] -> w592
          tunnel: w581 -> [_ w607]
          tunnel: w588 -> [w595 w606]
          tunnel: [w595 w602] -> w586
          tunnel: [w594 w601] -> w585
          tunnel: w582 -> [_ w597]
          tunnel: w580 -> [_ w596]
          tunnel: w575 -> [w594 w598]
          frame False {
          }
          frame True {
            n210 = invoke class="Tree (strict)" method="Edit Tree Items.Move Item"(reference=w611, error in=w598, "tag"=w609, "New Parent"=w607) -> (error out=w599:errorcluster)  [unwired: 3 in, 6 out]
            n211 = Bundle By Name(cluster=T6 {"node ref"=refnum, "new parent"=refnum} ("Cluster"), "new parent"=w596, "node ref"=w597) -> (w605:T6)
            n212 = Flatten To String(anything=w605, error in (no error)=w599) -> (data string=w604:string, error out=w600:errorcluster)  [unwired: 2 in, 1 out]
            n213 = call <vilib>:"Send Local Message.vi"("message queue in"=w606, "message name"="Move", "message value"=w604, "error in"=w600) -> ("message queue out"=w602:T4, "error out"=w601:errorcluster)  [unwired: 9 in, 1 out]
          }
        }
        n214 = event-data("Accepted?"=w592) -> ()  [unwired: 1 in, 1 out]
      }
      event "Exit": Value Change {
        # "Exit the application                                           >> Stop this message generator loop    Cleaning errors if the other loop stop this one"
        n215 = event-data() -> ()  [unwired: 1 in, 1 out]
        n216 = call <vilib>:"Send Local Message.vi"("message queue in"=w616, "message name"="Close", "error in"=w614) -> ("message queue out"=w612:T4, "error out"=w617:errorcluster)  [unwired: 10 in, 1 out]
        n217 = call <vilib>:"Clear Errors.vi"("error in (no error)"=w617) -> ("error out"=w613:errorcluster)  [unwired: 5 in, 1 out]
      }
      event "View": Drag Starting? {
        n218 = event-data() -> ("Data"=w629:T12, "CtlRef"=w631:refnum<vi>, "Coords"=w630:T11)  [unwired: 1 in]
        n219 = invoke class="Tree (strict)" method="Point To Row Column"(reference=w631, error in=w622, "Point"=w630) -> (error out=w621:errorcluster, "Tag"=w628:string)  [unwired: 5 in, 6 out]
        n220 = call <vilib>:"IDtoNode.vi"("error in"=w621, "ID"=w628) -> ("error out"=w620:errorcluster, "invalid Id"=w627:bool, "node ref"=w626:T2)  [unwired: 7 in]
        n221 = case shown="False" w627 {
          tunnel: w626 -> [w639 _]
          tunnel: [w636 TRUE ("Removable")] -> w624
          tunnel: w620 -> [w635 w645]
          tunnel: [w632 w645] -> w619
          frame False {
            n222 = in-place {
              in-place-border: [w642] -> w638
              in-place-border: w635 -> [w641]
              in-place-border: [w640] -> w634
              n223 = in-place-dvr #9(w639) -> (w644:refnum<class "NISE_CEF_Node.lvclass">)  [unwired: 1 out]
              n224 = call-dynamic "EditOptions.vi"("error in"=w641, "node in"=w644) -> ("error out"=w640:errorcluster, "edit options"=w642:T13, "node out"=w643:refnum<class "NISE_CEF_Node.lvclass">)  [unwired: 6 in, 1 out]
              n225 = in-place-dvr #9(w643) -> (w633:errorcluster)  [unwired: 1 out]
            }
            n226 = Unbundle By Name(w638) -> ("movable"=w637:bool)
            n227 = Merge Errors(w633, w634) -> (w632:errorcluster)
            n228 = Not(x=w637) -> (.not. x?=w636:bool)
          }
          frame True {
          }
        }
        n229 = event-data("Data"=w629, "Drag Mode"=enum32{"copy or move", "copy only", "move only"}."move only", "Discard?"=w624) -> ()  [unwired: 1 in, 1 out]
      }
      event "View": Value Change {
        n230 = event-data() -> ("NewVal"=w650:string)  [unwired: 1 in]
        n231 = call <vilib>:"Send Local Message.vi"("message queue in"=w652, "message name"="ActivateNode" ("Message Name"), "message value"=w650, "error in"=w647) -> ("message queue out"=w649:T4, "error out"=w648:errorcluster)  [unwired: 9 in, 1 out]
      }
      event "View": event type 3.0.xa000003a {
        n232 = event-data() -> ("CtlRef"=w661:refnum<vi>, "Coords"=w658:T11)  [unwired: 1 in]
        n233 = invoke class="Tree (strict)" method="Point To Row Column"(reference=w661, error in=w655, "Point"=w658) -> (reference out=w660:refnum<vi>, error out=w654:errorcluster, "Tag"=w659:string)  [unwired: 5 in, 5 out]
        n234 = call <vilib>:"ValidDragDrop.vi"("error in"=w654, "drag over"=w659, "tree ref in"=w660) -> ("error out"=w653:errorcluster, "accepted"=w657:bool)  [unwired: 5 in, 2 out]
        n235 = event-data("Accepted?"=w657) -> ()  [unwired: 1 in, 1 out]
      }
      event Panel Close? {
        # "Intercepts the upper right close panel operation to allow a smooth shutdown as opposed to immediately killing the app."
        n236 = event-data() -> ()  [unwired: 1 in, 1 out]
        n237 = call <vilib>:"Send Local Message.vi"("message queue in"=w666, "message name"="Close?", "error in"=w663) -> ("message queue out"=w664:T4, "error out"=w662:errorcluster)  [unwired: 10 in, 1 out]
        n238 = event-data("Discard?"=TRUE) -> ()  [unwired: 1 in, 1 out]
      }
      event Menu Selection (User) {
        # "#USERCFG It is needed to add a Case for Every item on the menu"
        n239 = event-data() -> ("ItemTag"=w668:string, "ItemPath"=w673:string)  [unwired: 1 in]
        n240 = case shown="\"_File:_New\"" w673 {
          selector: w673 -> [_ _ _ _ _ w703]
          tunnel: w672 -> [w678 w683 w688 w693 w698 w711]
          tunnel: [w674 w679 w684 w689 w694 w708] -> w671
          tunnel: w670 -> [w676 w681 w686 w691 w696 w699]
          tunnel: [w675 w680 w685 w690 w695 w706] -> w669
          tunnel: w668 -> [_ _ _ _ _ w704]
          frame "_File:_New" {
            n241 = call <vilib>:"Send Local Message.vi"("message queue in"=w678, "message name"="New?" ("Message Name"), "error in"=w676) -> ("message queue out"=w674:T4, "error out"=w675:errorcluster)  [unwired: 10 in, 1 out]
          }
          frame "_File:_Open" {
            n242 = call <vilib>:"Send Local Message.vi"("message queue in"=w683, "message name"="Open?" ("Message Name"), "error in"=w681) -> ("message queue out"=w679:T4, "error out"=w680:errorcluster)  [unwired: 10 in, 1 out]
          }
          frame "_File:_Save" {
            n243 = call <vilib>:"Send Local Message.vi"("message queue in"=w688, "message name"="Save" ("Message Name"), "error in"=w686) -> ("message queue out"=w684:T4, "error out"=w685:errorcluster)  [unwired: 10 in, 1 out]
          }
          frame "_File:Save As..." {
            n244 = call <vilib>:"Send Local Message.vi"("message queue in"=w693, "message name"="SaveAs" ("Message Name"), "error in"=w691) -> ("message queue out"=w689:T4, "error out"=w690:errorcluster)  [unwired: 10 in, 1 out]
          }
          frame "_File:_Exit" {
            n245 = call <vilib>:"Send Local Message.vi"("message queue in"=w698, "message name"="Close?" ("Message Name"), "error in"=w696) -> ("message queue out"=w694:T4, "error out"=w695:errorcluster)  [unwired: 10 in, 1 out]
          }
          frame Default {
            n246 = Bundle("ItemTag"=w704, w703) -> (w702:cluster{"ItemTag":string, string})  [unwired: 1 in]
            n247 = Flatten To String(anything=w702, error in (no error)=w699) -> (data string=w701:string, error out=w700:errorcluster)  [unwired: 2 in, 1 out]
            n248 = call <vilib>:"Send Local Message.vi"("message queue in"=w711, "message name"="CleansubPanel", "error in"=w700) -> ("message queue out"=w710:T4, "error out"=w707:errorcluster)  [unwired: 10 in, 1 out]
            n249 = call <vilib>:"Send Local Message.vi"("message queue in"=w710, "message name"="CustomFileMenu" ("Message Name"), "message value"=w701, "error in"=w707) -> ("message queue out"=w708:T4, "error out"=w706:errorcluster)  [unwired: 9 in, 1 out]
          }
        }
      }
    }
    n250 = call "Error.vi"("error in (no error)"=w496, "message queue in"=w497) -> ()  [unwired: 9 in, 1 out]
  }
